vi "Module Loop.vi"(8 "error in (no error)":errorcluster, 11 "Messaging Server Module in":refnum<class "Messaging Server Module.lvclass">) -> (0 "error out":errorcluster, 3 "Messaging Server Module out":refnum<class "Messaging Server Module.lvclass">)   [LabVIEW 2020, in "Volatus.lvlib" / "Messaging Server Module.lvclass"]
uses:
  Messaging Server Module.lvclass
  Messaging Server Module.lvclass/Messaging Server Module.ctl
  Module/Module.lvclass
  Messaging Client/Messaging Server Client.lvclass
  Msg Client State.ctl
  Volatus.lvlib
  lv-vecto/Vecto/IP Resolver/IP Resolver.lvclass
  lv-vecto/Vecto/proto/TcpClientHello/Data.ctl
  lv-vecto/Vecto/proto/TcpClientHello/TcpClientHello.lvlib
  Messaging Client/Client Handshake.ctl
  C:/dev/lv20CE/relink/lv-volatus/Volatus/Module/Module.lvclass
  C:/dev/lv20CE/relink/lv-volatus/Volatus/Messaging Server Module/Messaging Server Module.lvclass
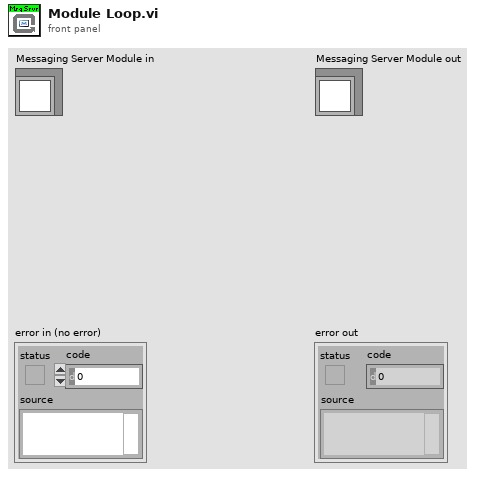
[diagram p1: front panel]
types:
  T1 = enum32{"Invalid", "Standard", "Closed", "Hidden", "Minimized", "Maximized"}
  T2 = typedef "Volatus.lvlib/Messaging Server Client.lvclass/Client Handshake.ctl" = cluster{"Endpoint":string, "TcpClientHello":T3}
  T3 = typedef "TcpClientHello.lvlib/Data.ctl" = cluster{"node_id":u32, "system":string, "cluster":string, "node_name":string, "app_version":string, "config_version":string, "config_hash":string, "node_alias":string}
  T4 = typedef "Volatus.lvlib/Msg Client State.ctl" = enum16{"Unknown", "Handshake", "Connected", "Closing"}
  T5 = typedef "Volatus.lvlib/Messaging Server Module.lvclass/Client Info.ctl" = cluster{"MsgQ":refnum<class "MessageQ.lvclass">, "Address":string, "Port":u16, "Client State":T4, "Last Update":dbl, "TCP":refnum<k5>, "Details":T6}
  T6 = typedef "TcpClientInfo.lvlib/Data.ctl" = cluster{"node_id":u32, "node_name":string, "app_version":string, "config_version":string, "config_hash":string, "node_alias":string, "address":string}
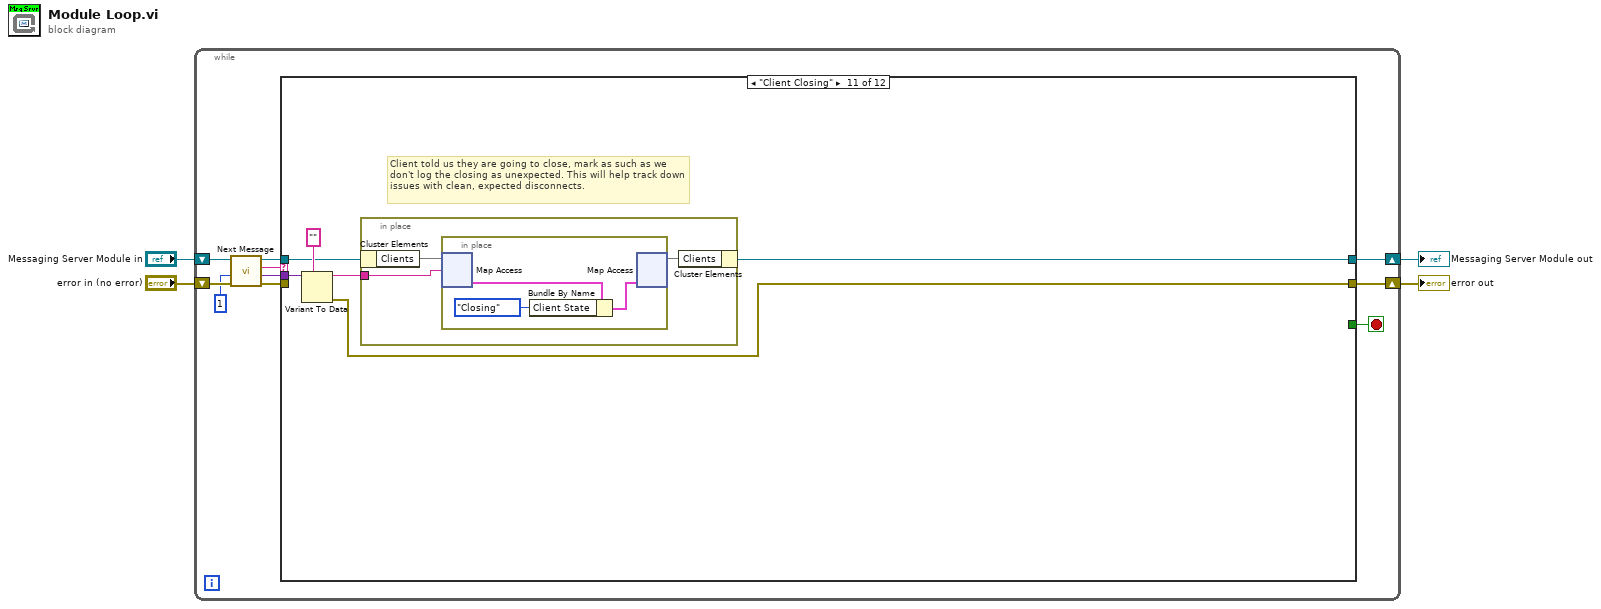
[diagram p0: block diagram]
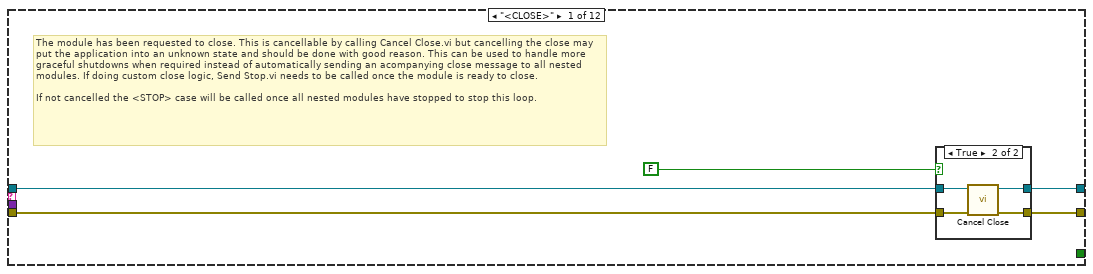
[diagram p2: hidden frame]
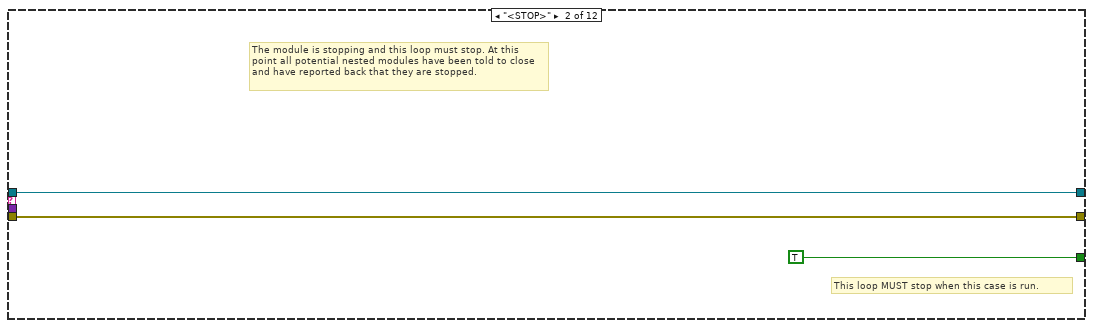
[diagram p4: hidden frame]
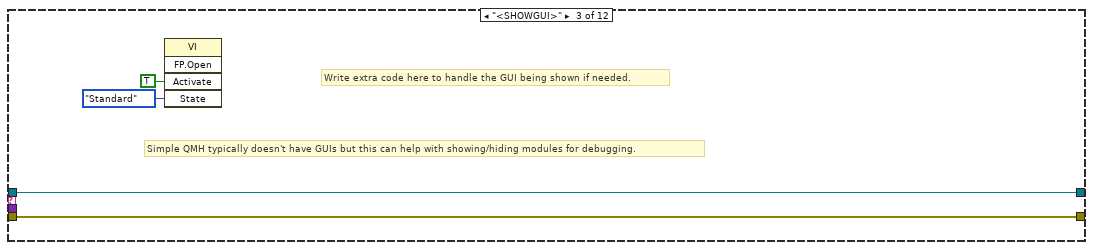
[diagram p5: hidden frame]
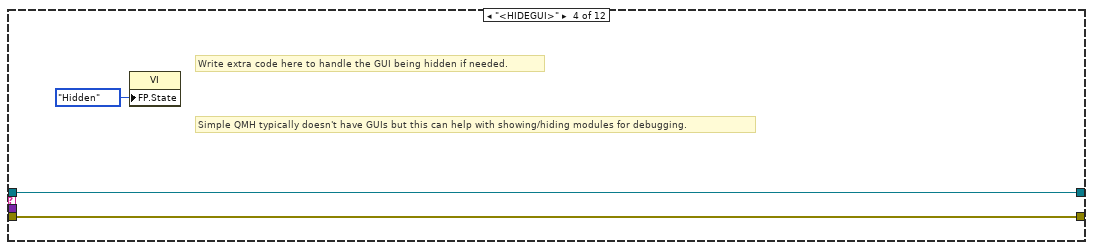
[diagram p6: hidden frame]
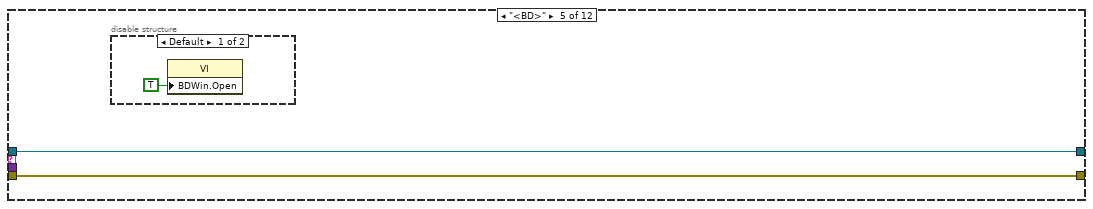
[diagram p7: hidden frame]
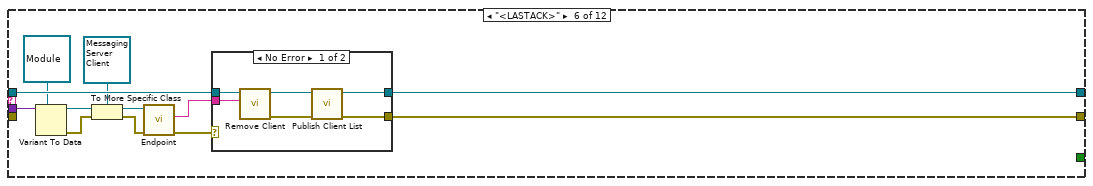
[diagram p9: hidden frame]
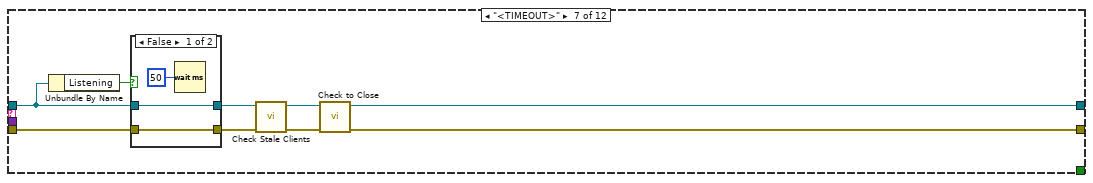
[diagram p11: hidden frame]
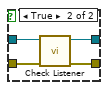
[diagram p12: hidden frame]
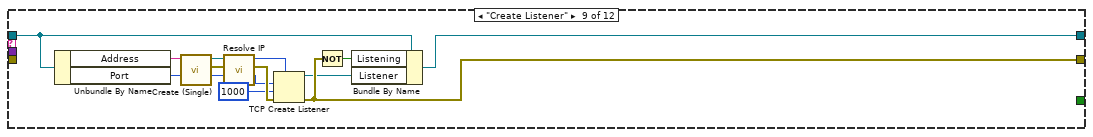
[diagram p14: hidden frame]
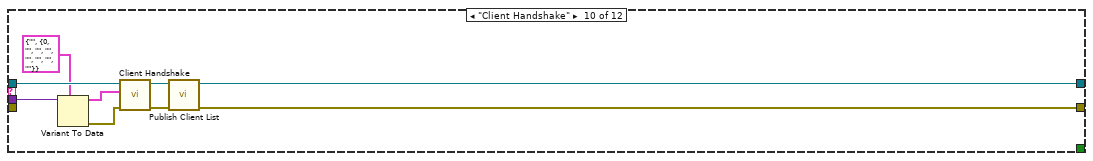
[diagram p15: hidden frame]
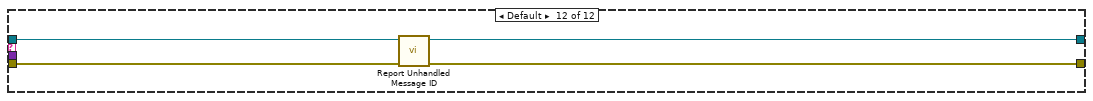
[diagram p16: hidden frame]
diagram:
  n1 = while {
    shift-right: [w9] -> w2
    shift-left: "Messaging Server Module in" -> [w14]
    shift-right: [w8] -> w1
    shift-left: "error in (no error)" -> [w13]
    stop <- w7 stop-if-true
    n2 = call "Next Message.vi"("error in (no error)"=w13, "Timeout ms (-1)"=1, "Module in"=w14) -> ("error out"=w12:errorcluster, "Data"=w6:variant, "ID"=w11:string, "Module out"=w10:refnum<class "Messaging Server Module.lvclass">)  [unwired: 5 in]
    n3 = case shown="\"Client Closing\"" w11 {
      tunnel: w12 -> [w19 w27 w31 w34 w36 _ w67 w75 _ _ _ w113]
      tunnel: w10 -> [w17 w28 w32 w35 w37 w50 w60 w76 w86 w97 w101 w111]
      tunnel: [w16 w28 w32 w35 w37 w42 w64 w76 w79 w89 w99 w110] -> w9
      tunnel: [w18 w27 w31 w34 w36 w40 w65 w75 w88 w91 w98 w112] -> w8
      tunnel: [_ TRUE _ _ _ _ _ _ _ _ _ _] -> w7
      tunnel: w6 -> [_ _ _ _ _ w49 _ _ _ w96 w103 _]
      frame "<CLOSE>" {
        # "The module has been requested to close. This is cancellable by calling Cancel Close.vi but cancelling the close may put the application into an unknown state and should be done with good reason. This can be used to handle more graceful shutdowns when required instead of automatically sending an acompanying close message to all nested modules. If doing custom close logic, Send Stop.vi needs to be called once the module is ready to close.\n\nIf not cancelled the <STOP> case will be called once all nested modules have stopped to stop this loop."
        n4 = case shown="True" FALSE {
          tunnel: w19 -> [w20 w25]
          tunnel: [w20 w24] -> w18
          tunnel: w17 -> [w21 w23]
          tunnel: [w21 w22] -> w16
          frame False {
          }
          frame True {
            n5 = call "Cancel Close.vi"("error in (no error)"=w25, "Module in"=w23) -> ("error out"=w24:errorcluster, "Module out"=w22:refnum<class "Messaging Server Module.lvclass">)  [unwired: 8 in]
          }
        }
      }
      frame "<STOP>" {
        # "This loop MUST stop when this case is run."
        # "The module is stopping and this loop must stop. At this point all potential nested modules have been told to close and have reported back that they are stopped."
      }
      frame "<SHOWGUI>" {
        # "Simple QMH typically doesn't have GUIs but this can help with showing/hiding modules for debugging."
        # "Write extra code here to handle the GUI being shown if needed."
        n6 = invoke class="VI" method="FP.Open"("Activate"=TRUE ("Activate?"), "State"=T1."Standard") -> ()  [unwired: 3 in, 5 out]
      }
      frame "<HIDEGUI>" {
        # "Simple QMH typically doesn't have GUIs but this can help with showing/hiding modules for debugging."
        # "Write extra code here to handle the GUI being hidden if needed."
        n7 = property class="VI"("FP.State"=T1."Hidden" ("Front Panel Window:State")) -> ()  [unwired: 2 in, 2 out]
      }
      frame "<BD>" {
        n8 = disable-structure shown="Default" {
          frame condition #0 (active) {
            n9 = property class="VI"("BDWin.Open"=TRUE ("Block Diagram Window:Open")) -> ()  [unwired: 2 in, 2 out]
          }
          frame condition #1 {
          }
        }
      }
      frame "<LASTACK>" {
        n10 = Variant To Data(type=refnum<class "Module.lvclass"> refnum ("Volatus:Module"), Variant=w49) -> (data=w47:refnum<class "Module.lvclass">, error out=w46:errorcluster)  [unwired: 1 in]
        n11 = To More Specific Class(target class=refnum<class "Messaging Server Client.lvclass"> refnum ("Volatus:Messaging Client.lvclass"), reference=w47, error in=w46) -> (specific class reference=w44:refnum<class "Messaging Server Client.lvclass">, error out=w43:errorcluster)
        n12 = call "Endpoint.vi"("error in (no error)"=w43, "Messaging Client in"=w44) -> ("error out"=w39:errorcluster, "Endpoint"=w41:string)  [unwired: 7 in, 1 out]
        n13 = case shown="No Error" w39 {
          selector: w39 -> [_ w58]
          tunnel: w50 -> [w56 w57]
          tunnel: [w51 w57] -> w42
          tunnel: w41 -> [w55 _]
          tunnel: [w53 w58] -> w40
          frame No Error {
            n14 = call "Remove Client.vi"("Endpoint"=w55, "Messaging Server Module in"=w56) -> ("error out"=w54:errorcluster, "Messaging Server Module out"=w52:refnum<class "Messaging Server Module.lvclass">)  [unwired: 8 in]
            n15 = call "Publish Client List.vi"("error in (no error)"=w54, "Messaging Server Module in"=w52) -> ("error out"=w53:errorcluster, "Messaging Server Module out"=w51:refnum<class "Messaging Server Module.lvclass">)  [unwired: 8 in]
          }
          frame Error {
          }
        }
      }
      frame "<TIMEOUT>" {
        n16 = Unbundle By Name(w60) -> ("Listening"=w59:bool)
        n17 = case shown="False" w59 {
          tunnel: w67 -> [w69 w74]
          tunnel: [w69 w73] -> w66
          tunnel: [w70 w72] -> w62
          tunnel: w60 -> [w70 w71]
          frame False {
            n18 = Wait (ms)(milliseconds to wait=u32 50) -> ()  [unwired: 1 out]
          }
          frame True {
            n19 = call "Check Listener.vi"("error in (no error)"=w74, "Messaging Server Module in"=w71) -> ("error out"=w73:errorcluster, "Messaging Server Module out"=w72:refnum<class "Messaging Server Module.lvclass">)  [unwired: 8 in]
          }
        }
        n20 = call "Check Stale Clients.vi"("error in (no error)"=w66, "Messaging Server Module in"=w62) -> ("error out"=w63:errorcluster, "Messaging Server Module out"=w61:refnum<class "Messaging Server Module.lvclass">)  [unwired: 8 in]
        n21 = call "Check to Close.vi"("error in (no error)"=w63, "Messaging Server Module in"=w61) -> ("error out"=w65:errorcluster, "Messaging Server Module out"=w64:refnum<class "Messaging Server Module.lvclass">)  [unwired: 8 in]
      }
      frame "Initialize" {
      }
      frame "Create Listener" {
        n22 = Unbundle By Name(w86) -> ("Address"=w85:string, "Port"=w82:u16)
        n23 = call "Create (Single).vi"("Binding"=w85) -> ("error out"=w80:errorcluster, "IP Resolver"=w84:refnum<class "IP Resolver.lvclass">)  [unwired: 9 in]
        n24 = call "Resolve IP.vi"("error in (no error)"=w80, "IP Resolver in"=w84) -> ("error out"=w87:errorcluster, "U32 Address"=w83:u32)  [unwired: 8 in]
        n25 = TCP Create Listener(7:w83, 8:w87, 9:1000 ("timeout ms (25000)"), 10:w82) -> (0:w88:errorcluster, 3:w78:refnum<k5>)  [unwired: 1 in, 1 out]
        n26 = Not(x=w88) -> (.not. x?=w77:bool)
        n27 = Bundle By Name(cluster=w86, "Listening"=w77, "Listener"=w78) -> (w79:refnum<class "Messaging Server Module.lvclass">)
      }
      frame "Client Handshake" {
        n28 = Variant To Data(type=T2 {"Endpoint"="", "TcpClientHello"={"node_id"=0, "system"="", "cluster"="", "node_name"="", "app_version"="", "config_version"="", "config_hash"="", "node_alias"=""}} ("Client Handshake"), Variant=w96) -> (data=w94:T2, error out=w93:errorcluster)  [unwired: 1 in]
        n29 = call "Client Handshake.vi"("error in (no error)"=w93, "Client Handshake"=w94, "Messaging Server Module in"=w97) -> ("error out"=w92:errorcluster, "Messaging Server Module out"=w90:refnum<class "Messaging Server Module.lvclass">)  [unwired: 7 in]
        n30 = call "Publish Client List.vi"("error in (no error)"=w92, "Messaging Server Module in"=w90) -> ("error out"=w91:errorcluster, "Messaging Server Module out"=w89:refnum<class "Messaging Server Module.lvclass">)  [unwired: 8 in]
      }
      frame "Client Closing" {
        # "Client told us they are going to close, mark as such as we don't log the closing as unexpected. This will help track down issues with clean, expected disconnects."
        n31 = Variant To Data(type="", Variant=w103) -> (data=w100:string, error out=w98:errorcluster)  [unwired: 1 in]
        n32 = in-place {
          in-place-border: w100 -> [w105]
          n33 = in-place-cluster #1(w101) -> ("Clients"=w106:map{string, T5})
          n34 = in-place {
            n35 = in-place-map #2(w106, w105) -> (w109:T5)  [unwired: 1 in, 1 out]
            n36 = Bundle By Name(cluster=w109, "Client State"=Msg_Client_State."Closing") -> (w107:T5)
            n37 = in-place-map #2(w107) -> (w104:map{string, T5})  [unwired: 1 in, 2 out]
          }
          n38 = in-place-cluster #1("Clients"=w104) -> (w99:refnum<class "Messaging Server Module.lvclass">)
        }
      }
      frame Default {
        n39 = call "Report Unhandled Message ID.vi"("error in (no error)"=w113, "Module in"=w111) -> ("error out"=w112:errorcluster, "Module out"=w110:refnum<class "Messaging Server Module.lvclass">)  [unwired: 8 in]
      }
    }
  }
  "error out" <- w1
  "Messaging Server Module out" <- w2
